vi "Set.vi"(6 "error":errorcluster, 7 "Input Command String":string, 8 "Quantity":string(combo), 9 "VISA resource name":refnum<visa-resource-name>) -> (0 "error out":errorcluster, 2 "Returned":dbl format="%_4f", 3 "VISA resource name out":refnum<visa-resource-name>, 5 "Response":string)   [LabVIEW 2018, in "BigSkyControl.lvlib"]
uses:
  BigSkyControl.lvlib
panel:
  out "Read return count":u32
  in  "byte count":u32=1024
  out "Write return count":u32
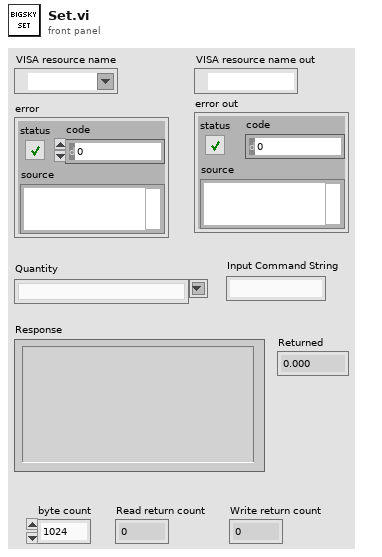
[diagram p1: front panel]
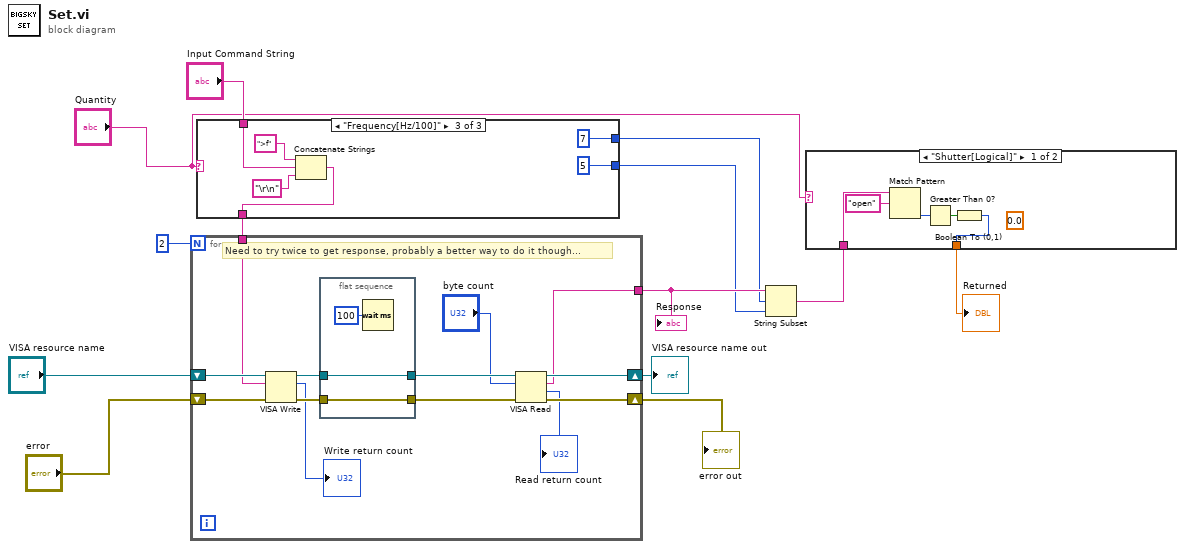
[diagram p0: block diagram]
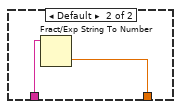
[diagram p2: hidden frame]
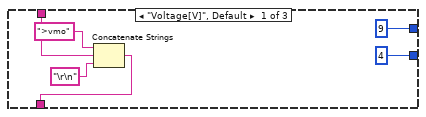
[diagram p3: hidden frame]
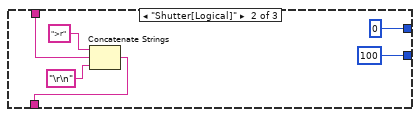
[diagram p4: hidden frame]
diagram:
  n1 = case shown="\"Frequency[Hz/100]\"" "Quantity" {
    tunnel: [w14 w20 w26] -> w7
    tunnel: [9 ("offset (0)") 0 ("offset (0)") 7 ("offset (0)")] -> w6
    tunnel: [4 ("length (rest)") 100 ("length (rest)") 5 ("length (rest)")] -> w5
    tunnel: "Input Command String" -> [w15 w21 w27]
    frame "Voltage[V]", Default {
      n2 = Concatenate Strings(">vmo" ("string"), w15, "\r\n" ("write buffer")) -> (w14:string)
    }
    frame "Shutter[Logical]" {
      n3 = Concatenate Strings(">r" ("string"), w21, "\r\n" ("write buffer")) -> (w20:string)
    }
    frame "Frequency[Hz/100]" {
      n4 = Concatenate Strings(">f" ("string"), w27, "\r\n" ("write buffer")) -> (w26:string)
    }
  }
  n5 = for {
    N: 2 -> [_]
    shift-right: [w43] -> w10
    shift-left: "VISA resource name" -> [w42]
    shift-right: [w44] -> w9
    shift-left: "error" -> [w41]
    tunnel: [w33] -> w8
    tunnel: w7 -> [w32]
    # "Need to try twice to get response, probably a better way to do it though..."
    n6 = VISA Write(VISA resource name=w42, write buffer=w32, error in (no error)=w41) -> (VISA resource name out=w39:refnum<visa-resource-name>, return count=→"Write return count":u32, error out=w40:errorcluster)
    n7 = flat-sequence {
      tunnel: w40 -> [w47]
      tunnel: [w47] -> w37
      tunnel: w39 -> [w46]
      tunnel: [w46] -> w38
      frame #0 {
        n8 = Wait (ms)(milliseconds to wait=u32 100) -> ()  [unwired: 1 out]
      }
    }
    n9 = VISA Read(VISA resource name=w38, byte count="byte count", error in (no error)=w37) -> (VISA resource name out=w43:refnum<visa-resource-name>, read buffer=w33:string, return count=→"Read return count":u32, error out=w44:errorcluster)
  }
  "Response" <- w8
  "VISA resource name out" <- w10
  "error out" <- w9
  n10 = String Subset(string=w8, offset (0)=w6, length (rest)=w5) -> (substring=w2:string)
  n11 = case shown="\"Shutter[Logical]\"" "Quantity" {
    tunnel: w2 -> [w52 w54]
    tunnel: [w48 w53] -> w1
    frame "Shutter[Logical]" {
      (unwired) 0.0
      n12 = Match Pattern(string=w52, regular expression="open") -> (offset past match=w50:i32)  [unwired: 1 in, 3 out]
      n13 = Greater Than 0?(x=w50) -> (x > 0?=w49:bool)
      n14 = Boolean To (0,1)(Boolean=w49) -> (0, 1=w48:i16)
    }
    frame Default {
      n15 = Fract/Exp String To Number(string=w54) -> (number=w53:dbl)  [unwired: 3 in, 1 out]
    }
  }
  "Returned" <- w1
